vi "ArduinoReader.vi"() -> ()   [LabVIEW 2014]
uses:
  <vilib>/Instr/_visa.llb/VISA Configure Serial Port (Instr).vi
  <vilib>/regexp/Match Regular Expression.xnode
panel:
  in  "name":string="127.0.0.1"
  in  "Reset COM":bool
  out "Serial Communication Error":errorcluster
  in  "COM Port":refnum<visa-resource-name>
  out "Last Arduino Communication":timestamp
  out "Message":string
  out "Message Number":i32
  out "RPM":dbl
  out "Error Count":i32
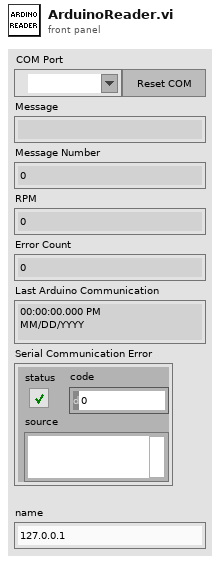
[diagram p1: front panel]
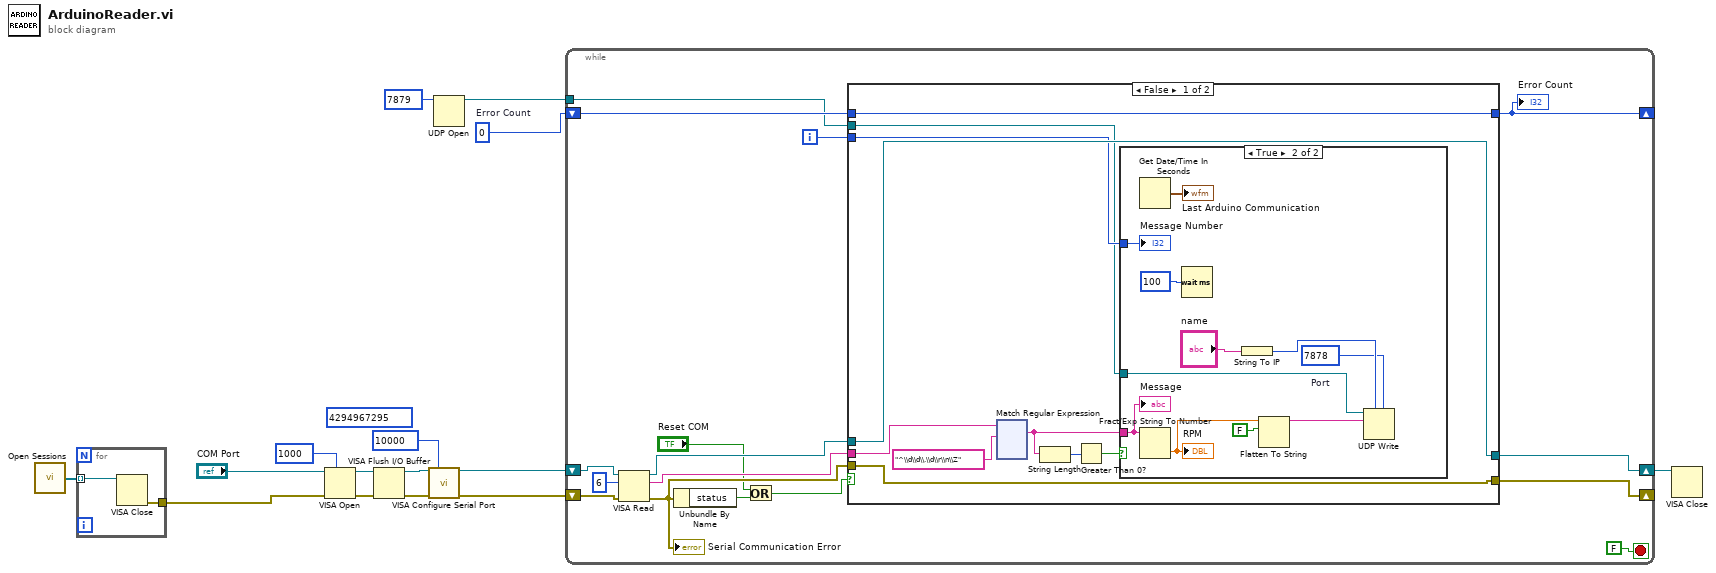
[diagram p0: block diagram]
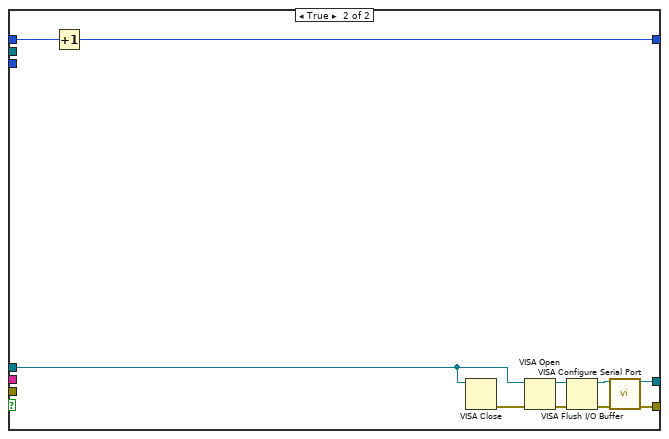
[diagram p3: hidden frame]
diagram:
  (unwired) u32 4294967295 ("timeout (10sec)")
  w10 = 0  # Error Count
  n1 = call <vilib>:"Open Sessions.vi"() -> ("Array of Refnums"=w12:refnum<visa-resource-name>[])  [unwired: 2 in]
  n2 = for {
    tunnel: w12 -> [w17] mode=indexing
    tunnel: [w16] -> w11
    n3 = VISA Close(VISA resource name=w17) -> (error out=w16:errorcluster)  [unwired: 1 in]
  }
  n4 = VISA Open(timeout (0)=u32 1000 ("VISA Open timeout (0)"), error in (no error)=w11, VISA resource name="COM Port") -> (VISA resource name=w13:refnum<visa-resource-name>, error out=w9:errorcluster)  [unwired: 2 in]
  n5 = VISA Flush I/O Buffer(VISA resource name=w13, error in (no error)=w9) -> (VISA resource name out=w15:refnum<visa-resource-name>, error out=w8:errorcluster)  [unwired: 1 in]
  n6 = call-poly "VISA Configure Serial Port"("VISA resource name"=w15, "timeout (10sec)"=u32 10000, "error in (no error)"=w8) -> ("VISA resource name out"=w5:refnum<visa-resource-name>, "error out"=w4:errorcluster)  [unwired: 11 in]
  n7 = UDP Open(11:u16 7879 ("port")) -> (port=w7:refnum<k16>)  [unwired: 4 in, 2 out]
  n8 = while {
    shift-right: [w28] -> w14
    shift-left: w5 -> [w33]
    shift-right: [w30] -> _
    shift-left: w10 -> [w31]
    shift-right: [w24] -> _
    shift-left: w4 -> [w25]
    tunnel: w7 -> [w18]
    i -> [w26]
    stop <- FALSE stop-if-true
    n9 = VISA Read(VISA resource name=w33, byte count=u32 6, error in (no error)=w25) -> (VISA resource name out=w29:refnum<visa-resource-name>, read buffer=w27:string, error out=w22:errorcluster)  [unwired: 1 out]
    "Serial Communication Error" <- w22
    n10 = Unbundle By Name(w22) -> ("status"=w19:bool)
    n11 = Or(x="Reset COM", y=w19) -> (x .or. y?=w21:bool)
    n12 = case shown="False" w21 {
      tunnel: w31 -> [w43 w178]
      tunnel: [w43 w177] -> w30
      tunnel: w29 -> [w42 w172]
      tunnel: [w42 w173] -> w28
      tunnel: w27 -> [w37 _]
      tunnel: w26 -> [w36 _]
      tunnel: [w35 w169] -> w24
      tunnel: w22 -> [w35 _]
      tunnel: w18 -> [w34 _]
      frame False {
        n13 = xnode "Match Regular Expression"("input string"=w37, "regular expression"="^\\d\\d\\.\\d\\r\\n\\Z") -> ("whole match"=w40:string)  [unwired: 4 in, 4 out]
        n14 = String Length(string=w40) -> (length=w38:i32)
        n15 = Greater Than 0?(x=w38) -> (x > 0?=w39:bool)
        n16 = case shown="True" w39 {
          tunnel: w40 -> [_ w53]
          tunnel: w36 -> [_ w54]
          tunnel: w34 -> [_ w48]
          frame False {
          }
          frame True {
            w46 = u16 7878  # Port
            n17 = Get Date/Time In Seconds() -> (seconds since 1Jan1904=→"Last Arduino Communication":timestamp)
            n18 = Fract/Exp String To Number(string=w53) -> (number=w50:dbl)  [unwired: 3 in, 1 out]
            "RPM" <- w50
            n19 = Wait (ms)(milliseconds to wait=u32 100) -> ()  [unwired: 1 out]
            n20 = String To IP(1:"name") -> (0:w47:u32)
            n21 = Flatten To String(anything=w50, prepend array or string size? (T)=FALSE) -> (data string=w49:string)  [unwired: 2 in, 2 out]
            n22 = UDP Write(address=w47, port or service name=w46, connection ID=w48, data in=w49) -> ()  [unwired: 2 in, 2 out]
            "Message" <- w53
            "Message Number" <- w54
          }
        }
      }
      frame True {
        n23 = Increment(x=w178) -> (x+1=w177:i32)
        n24 = VISA Close(VISA resource name=w172) -> (error out=w176:errorcluster)  [unwired: 1 in]
        n25 = VISA Open(error in (no error)=w176, VISA resource name=w172) -> (VISA resource name=w175:refnum<visa-resource-name>, error out=w171:errorcluster)  [unwired: 3 in]
        n26 = VISA Flush I/O Buffer(VISA resource name=w175, error in (no error)=w171) -> (VISA resource name out=w174:refnum<visa-resource-name>, error out=w170:errorcluster)  [unwired: 1 in]
        n27 = call-poly "VISA Configure Serial Port"("VISA resource name"=w174, "error in (no error)"=w170) -> ("VISA resource name out"=w173:refnum<visa-resource-name>, "error out"=w169:errorcluster)  [unwired: 12 in]
      }
    }
    "Error Count" <- w30
  }
  n28 = VISA Close(VISA resource name=w14) -> ()  [unwired: 1 in, 1 out]
